vi "c Spark Set Parameter Float32.vi"(8 "error in (no error)":errorcluster, 9 "value":sgl, 10 "paramID":T1, 11 "handle":T2) -> (0 "error out":errorcluster, 2 "function return":T3, 3 "handle out":T2)   [LabVIEW 2023, in "REVLibDriver.lvlib"]
doc: "c_REVLib_ErrorCode c_Spark_SetParameterFloat32(c_Spark_handle handle,\n c_Spark_ConfigParameter paramId,\n float value);"
uses:
  REVLibDriver.lvlib
  REVLibDriver.dll
  Custom Controls/c_Spark_handle.ctl
  subvi/RevLibError.ctl
  Custom Controls/c_Spark_ConfigParameter.ctl
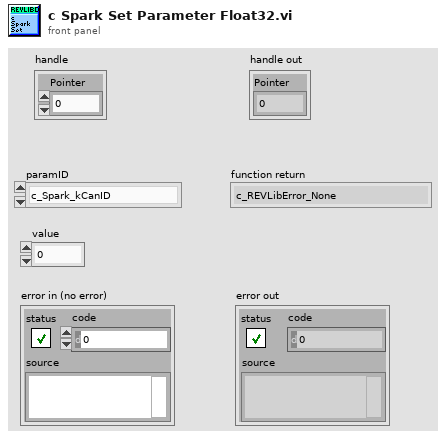
[diagram p1: front panel]
types:
  T1 = typedef "REVLibDriver.lvlib/c_Spark_ConfigParameter.ctl" = enum16{"c_Spark_kCanID", "c_Spark_kInputMode", "c_Spark_kMotorType", "c_Spark_kCommAdvance", "c_Spark_kSensorType", "c_Spark_kCtrlType", "c_Spark_kIdleMode", "c_Spark_kInputDeadband", "c_Spark_kFeedbackSensorPID0", "c_Spark_kFeedbackSensorPID1", "c_Spark_kPolePairs", "c_Spark_kCurrentChop", "c_Spark_kCurrentChopCycles", "c_Spark_kP_0", "c_Spark_kI_0", "c_Spark_kD_0", "c_Spark_kF_0", "c_Spark_kIZone_0", "c_Spark_kDFilter_0", "c_Spark_kOutputMin_0", "c_Spark_kOutputMax_0", "c_Spark_kP_1", "c_Spark_kI_1", "c_Spark_kD_1", "c_Spark_kF_1", "c_Spark_kIZone_1", "c_Spark_kDFilter_1", "c_Spark_kOutputMin_1", "c_Spark_kOutputMax_1", "c_Spark_kP_2", "c_Spark_kI_2", "c_Spark_kD_2", "c_Spark_kF_2", "c_Spark_kIZone_2", "c_Spark_kDFilter_2", "c_Spark_kOutputMin_2", "c_Spark_kOutputMax_2", "c_Spark_kP_3", "c_Spark_kI_3", "c_Spark_kD_3", "c_Spark_kF_3", "c_Spark_kIZone_3", "c_Spark_kDFilter_3", "c_Spark_kOutputMin_3", "c_Spark_kOutputMax_3", "c_Spark_kInverted", "c_Spark_kOutputRatio", "c_Spark_kSerialNumberLow", "c_Spark_kSerialNumberMid", "c_Spark_kSerialNumberHigh", "c_Spark_kLimitSwitchFwdPolarity", "c_Spark_kLimitSwitchRevPolarity", "c_Spark_kHardLimitFwdEn", "c_Spark_kHardLimitRevEn", "c_Spark_kSoftLimitFwdEn", "c_Spark_kSoftLimitRevEn", "c_Spark_kRampRate", "c_Spark_kFollowerID", "c_Spark_kFollowerConfig", "c_Spark_kSmartCurrentStallLimit", "c_Spark_kSmartCurrentFreeLimit", "c_Spark_kSmartCurrentConfig", "c_Spark_kSmartCurrentReserved", "c_Spark_kMotorKv", "c_Spark_kMotorR", "c_Spark_kMotorL", "c_Spark_kMotorRsvd1", "c_Spark_kMotorRsvd2", "c_Spark_kMotorRsvd3", "c_Spark_kEncoderCountsPerRev", "c_Spark_kEncoderAverageDepth", "c_Spark_kEncoderSampleDelta", "c_Spark_kEncoderInverted", "c_Spark_kEncoderRsvd1", "c_Spark_kVoltageCompMode", "c_Spark_kCompensatedNominalVoltage", "c_Spark_kSmartMotionMaxVelocity_0", "c_Spark_kSmartMotionMaxAccel_0", "c_Spark_kSmartMotionMinVelOutput_0", "c_Spark_kSmartMotionAllowedClosedLoopError_0", "c_Spark_kSmartMotionAccelStrategy_0", "c_Spark_kSmartMotionMaxVelocity_1", "c_Spark_kSmartMotionMaxAccel_1", "c_Spark_kSmartMotionMinVelOutput_1", "c_Spark_kSmartMotionAllowedClosedLoopError_1", "c_Spark_kSmartMotionAccelStrategy_1", "c_Spark_kSmartMotionMaxVelocity_2", "c_Spark_kSmartMotionMaxAccel_2", "c_Spark_kSmartMotionMinVelOutput_2", "c_Spark_kSmartMotionAllowedClosedLoopError_2", "c_Spark_kSmartMotionAccelStrategy_2", "c_Spark_kSmartMotionMaxVelocity_3", "c_Spark_kSmartMotionMaxAccel_3", "c_Spark_kSmartMotionMinVelOutput_3", "c_Spark_kSmartMotionAllowedClosedLoopError_3", "c_Spark_kSmartMotionAccelStrategy_3", "c_Spark_kIMaxAccum_0", "c_Spark_kSlot3Placeholder1_0", "c_Spark_kSlot3Placeholder2_0", "c_Spark_kSlot3Placeholder3_0", "c_Spark_kIMaxAccum_1", "c_Spark_kSlot3Placeholder1_1", "c_Spark_kSlot3Placeholder2_1", "c_Spark_kSlot3Placeholder3_1", "c_Spark_kIMaxAccum_2", "c_Spark_kSlot3Placeholder1_2", "c_Spark_kSlot3Placeholder2_2", "c_Spark_kSlot3Placeholder3_2", "c_Spark_kIMaxAccum_3", "c_Spark_kSlot3Placeholder1_3", "c_Spark_kSlot3Placeholder2_3", "c_Spark_kSlot3Placeholder3_3", "c_Spark_kPositionConversionFactor", "c_Spark_kVelocityConversionFactor", "c_Spark_kClosedLoopRampRate", "c_Spark_kSoftLimitFwd", "c_Spark_kSoftLimitRev", "c_Spark_kSoftLimitRsvd0", "c_Spark_kSoftLimitRsvd1", "c_Spark_kAnalogRevPerVolt", "c_Spark_kAnalogRotationsPerVoltSec", "c_Spark_kAnalogAverageDepth", "c_Spark_kAnalogSensorMode", "c_Spark_kAnalogInverted", "c_Spark_kAnalogSampleDelta", "c_Spark_kAnalogRsvd0", "c_Spark_kAnalogRsvd1", "c_Spark_kDataPortConfig", "c_Spark_kAltEncoderCountsPerRev", "c_Spark_kAltEncoderAverageDepth", "c_Spark_kAltEncoderSampleDelta", "c_Spark_kAltEncoderInverted", "c_Spark_kAltEncodePositionFactor", "c_Spark_kAltEncoderVelocityFactor", "c_Spark_kAltEncoderRsvd0", "c_Spark_kAltEncoderRsvd1", "c_Spark_kHallSensorSampleRate", "c_Spark_kHallSensorAverageDepth", "c_Spark_kNumParameters", "c_Spark_kDutyCyclePositionFactor", "c_Spark_kDutyCycleVelocityFactor", "c_Spark_kDutyCycleInverted", "c_Spark_kDutyCycleSensorMode", "c_Spark_kDutyCycleAverageDepth", "c_Spark_kDutyCycleSampleDelta", "c_Spark_kDutyCycleOffsetv1p6p2", "c_Spark_kDutyCycleRsvd0", "c_Spark_kDutyCycleRsvd1", "c_Spark_kDutyCycleRsvd2", "c_Spark_kPositionPIDWrapEnable", "c_Spark_kPositionPIDMinInput", "c_Spark_kPositionPIDMaxInput", "c_Spark_kDutyCycleZeroCentered", "c_Spark_kDutyCyclePrescaler", "c_Spark_kDutyCycleOffset", "c_Spark_kProductId", "c_Spark_kDeviceMajorVersion", "c_Spark_kDeviceMinorVersion", "c_Spark_kUnused158", "c_Spark_kUnused159", "c_Spark_kUnused160", "c_Spark_kUnused161", "c_Spark_kUnused162", "c_Spark_kUnused163", "c_Spark_kUnused164", "c_Spark_kUnused165", "c_Spark_kMAXMotionMaxVelocity_0", "c_Spark_kMAXMotionMaxAccel_0", "c_Spark_kMAXMotionMaxJerk_0", "c_Spark_kMAXMotionAllowedClosedLoopError_0", "c_Spark_kMAXMotionMode_0", "c_Spark_kMAXMotionMaxVelocity_1", "c_Spark_kMAXMotionMaxAccel_1", "c_Spark_kMAXMotionMaxJerk_1", "c_Spark_kMAXMotionAllowedClosedLoopError_1", "c_Spark_kMAXMotionMode_1", "c_Spark_kMAXMotionMaxVelocity_2", "c_Spark_kMAXMotionMaxAccel_2", "c_Spark_kMAXMotionMaxJerk_2", "c_Spark_kMAXMotionAllowedClosedLoopError_2", "c_Spark_kMAXMotionMode_2", "c_Spark_kMAXMotionMaxVelocity_3", "c_Spark_kMAXMotionMaxAccel_3", "c_Spark_kMAXMotionMaxJerk_3", "c_Spark_kMAXMotionAllowedClosedLoopError_3", "c_Spark_kMAXMotionMode_3", "c_Spark_NumParameters"}
  T2 = typedef "REVLibDriver.lvlib/c_Spark_handle.ctl" = cluster{"Pointer":u64}
  T3 = typedef "REVLibDriver.lvlib/RevLibError.ctl" = enum16{"c_REVLibError_None", "c_REVLibError_General", "c_REVLibError_CANTimeout", "c_REVLibError_NotImplemented", "c_REVLibError_HAL", "c_REVLibError_CantFindFirmware", "c_REVLibError_FirmwareTooOld", "c_REVLibError_FirmwareTooNew", "c_REVLibError_ParamInvalidID", "c_REVLibError_ParamMismatchType", "c_REVLibError_ParamAccessMode", "c_REVLibError_ParamInvalid", "c_REVLibError_ParamNotImplementedDeprecated", "c_REVLibError_FollowConfigMismatch", "c_REVLibError_Invalid", "c_REVLibError_SetpointOutOfRange", "c_REVLibError_Unknown", "c_REVLibError_CANDisconnected", "c_REVLibError_DuplicateCANId", "c_REVLibError_InvalidCANId", "c_REVLibError_SparkMaxDataPortAlreadyConfiguredDifferently", "c_REVLibError_SparkFlexBrushedWithoutDock", "c_REVLibError_InvalidBrushlessEncoderConfiguration", "c_REVLibError_FeedbackSensorIncompatibleWithDataPortConfig", "c_REVLibError_ParamInvalidChannel", "c_REVLibError_ParamInvalidValue", "c_REVLibError_CannotPersistParametersWhileEnabled", "c_REVLibError_NotReadyToReceiveCommand", "c_REVLibError_NumCodes"}
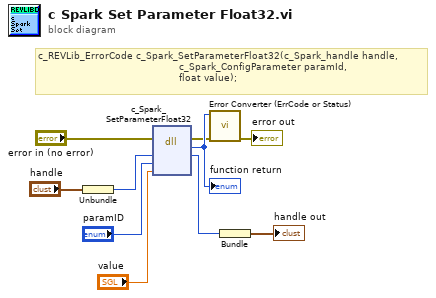
[diagram p0: block diagram]
diagram:
  # "c_REVLib_ErrorCode c_Spark_SetParameterFloat32(c_Spark_handle handle,\n                                               c_Spark_ConfigParameter paramId,\n                                               float value);"
  n1 = Unbundle("handle") -> ("Pointer"=w2:u64)
  n2 = dll-call lib="REVLibDriver.*" fn="c_Spark_SetParameterFloat32"(error in="error in (no error)", "handle"=w2, "paramId"="paramID", "value"="value") -> (error out=w4:errorcluster, "return type"=w10:u32, "handle"=w8:u64)  [unwired: 4 in, 1 out]
  "function return" <- w10
  n3 = call "Error Converter (ErrCode or Status).vi"("error in (no error)"=w4, "error code"=w10) -> ("error out"=→"error out":errorcluster)  [unwired: 9 in]
  n4 = Bundle("handle"=w8) -> (→"handle out":cluster{"handle":u64})  [unwired: 1 in]
